vi "Coord window-Column header entry window.vi"(11 "Column name in":string) -> (1 "Cancelled":bool, 3 "Column name out":string)   [LabVIEW 2013]
doc: "Use this template to create a dialog box with event handling."
uses:
  <vilib>/Utility/miscctls.llb/LVPointTypeDef.ctl
  Global Variables/General Globals.vi
panel:
  in  "Cancel":bool
  in  "OK":bool
  in  "Column name":string
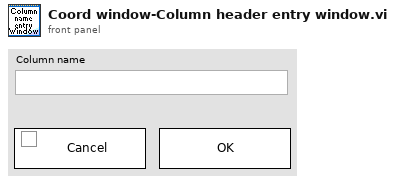
[diagram p1: front panel]
types:
  T1 = typedef "LVPointTypeDef.ctl" = cluster{"Horizontal":i16, "Vertical":i16}
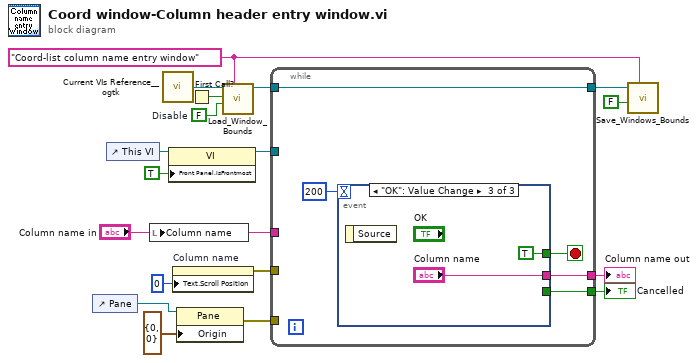
[diagram p0: block diagram]
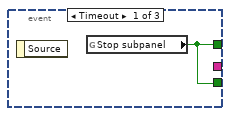
[diagram p2: hidden frame]
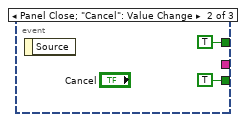
[diagram p3: hidden frame]
diagram:
  w7 = FALSE  # Disable
  w6 = "Coord-list column name entry window" ("Window Name (i.e. Key)")
  n1 = control-ref of="Pane"() -> (w11:refnum<vi>)
  n2 = control-ref of="This VI"() -> (w15:refnum<vi>)
  n3 = local write "Column name"("Column name in") -> ()
  n4 = call "Current VIs Reference__ogtk.vi"() -> ("Current VI's reference"=w9:refnum<vi>)  [unwired: 5 in]
  n5 = property on="Property Node" class="VI"(reference=w15, "Front Panel.IsFrontmost"=TRUE ("Front Panel Window:Is Frontmost")) -> (reference out=w14:refnum<vi>)  [unwired: 1 in, 1 out]
  n6 = property on="Column name" class="Str"("Text.Scroll Position"=u32 0) -> (error out=w17:errorcluster)  [unwired: 2 in, 1 out]
  n7 = property class="Pane"(reference=w11, "Origin"=T1 {"Horizontal"=0, "Vertical"=0}) -> (error out=w12:errorcluster)  [unwired: 1 in, 1 out]
  n8 = First Call?() -> (First Call?: T/F=w8:bool)
  n9 = call "Load_Window_Bounds.vi"("Window Name (i.e. Key)"=w6, "Disable"=w7, "First Call"=w8, "Window VI's Ref"=w9) -> ("reference out"=w4:refnum<vi>)  [unwired: 4 in, 3 out]
  n10 = while {
    tunnel: "Column name in" -> [_]
    tunnel: w17 -> [_]
    tunnel: w12 -> [_]
    tunnel: w14 -> [_]
    tunnel: [w21] -> w10
    tunnel: w4 -> [w20]
    tunnel: [w20] -> w3
    tunnel: [w19] -> w2
    stop <- w23 stop-if-true
    n11 = event shown="[2] \"OK\": Value Change" {
      selector: _ -> [_ _ _]
      dyn-events: _ -> [_ _ _]
      timeout: 200 -> [_ _ _]
      tunnel: [w24 TRUE ("Stop?") TRUE ("Stop?")] -> w23
      tunnel: [w24 TRUE ("Stop subpanel") _] -> w21
      tunnel: [_ _ "Column name"] -> w19
      event Timeout {
        n12 = event-data() -> ()  [unwired: 1 in, 1 out]
        n13 = global read "General Globals.vi" "Stop subpanel"() -> (w24:bool)
      }
      event Panel Close; "Cancel": Value Change {
        n14 = event-data() -> ()  [unwired: 1 in, 1 out]
      }
      event "OK": Value Change {
        n15 = event-data() -> ()  [unwired: 1 in, 1 out]
      }
    }
  }
  "Cancelled" <- w10
  "Column name out" <- w2
  n16 = call "Save_Windows_Bounds.vi"("Window Name (i.e. Key)"=w6, "Front Panel Window:Open"=FALSE, "Window VI's Ref"=w3) -> ()  [unwired: 8 in, 1 out]
